vi "LDA_Align_PN_8 point.vi"(1 "Align Probe Using":enum16{"Green Beams", "Blue Beams"}(ring), 2 "Use Specification Beam Half-Angle":bool) -> (0 "Beam Data":T2={"Vg1 (Green 1 dir. vect.)"=[0.059117350659853476, -0.996541267827751, 0.05840068807144843], "Vg2  (Green 2 dir. vect.)"=[-0.05232536310393669, -0.9971561380468801, -0.054237373935992664], "Vb1 (Blue 1 dir. vect.)"=[-0.052923229613528855, -0.9969242065933935, 0.057803616456121795], "Vb2 (Blue 1 dir. vect.)"=[0.05971521716944564, -0.9967731992812374, -0.05364030232066602], "Porb (Orb XYZ posn. forced coplanar)"=[2201.0738225655555, -1199.3737231995547, 269.758310600838], "Porb (Orb XYZ posn. - allow skew)"=[2200.796256301178, -1199.3740953152687, 270.0329332816893], "Orb posn. uncertainty, +/- dx, dy, dz"=[0.13878313218879157, 0.00018605785703584843, 0.13731134042564008], "Vp (Actual Probe dir. vect)"=[0.003406702197773746, -0.9999920168246164, 0.0020882210543692924], "Yaw (deg)"=89.80480953887573, "Pitch (deg)"=0.11964634006213794, "In-Plane Roll (deg)"=45.305328966424156, "Beam Half Angle (deg)"=4.544091484248422, "B1 Close P11"=[0.0, 0.0, 0.0], "B1 Far P12"=[2158.01, -491.04, 229.28], "B2 Close P22"=[2158.01, -491.04, 229.28], "B2 Far P21"=[2158.01, -491.04, 229.28], "Projected Roll (deg)"=0.0, "Green Velocity Vector"=[0.0, 0.0, 0.0], "Blue Velocity Vector"=[0.0, 0.0, 0.0], "Probe is facing...."="-", "Calculation Method"=""} {"Vp (Actual Probe dir. vect)" format="%#_6f"; "Vg2  (Green 2 dir. vect.)" format="%#_6f"; "Vg1 (Green 1 dir. vect.)" format="%#_6f"})   [LabVIEW 2011]
uses:
  Controls/LDA_Beam_Cluster.ctl
  Gen Trav/Route mapping/Axis.ctl
  Controls/Tunnel_Coordinates.ctl
  Controls/User_Specific_mode.ctl
  Gen Trav/Trav_mode.ctl
  Globals/LDA_meas_global_1.vi
  Globals/Trav_pos_global.vi
panel:
  out "8 Peaked positions":dbl[][](array[numeric])
  out "Peakup up inputs":dbl[][](array[numeric])
  out "Fixed Axis":T1
  out "png folder":path
  out "Taught point names":string[](array[string])
  out "Taught Positions":dbl[][](array[numeric])
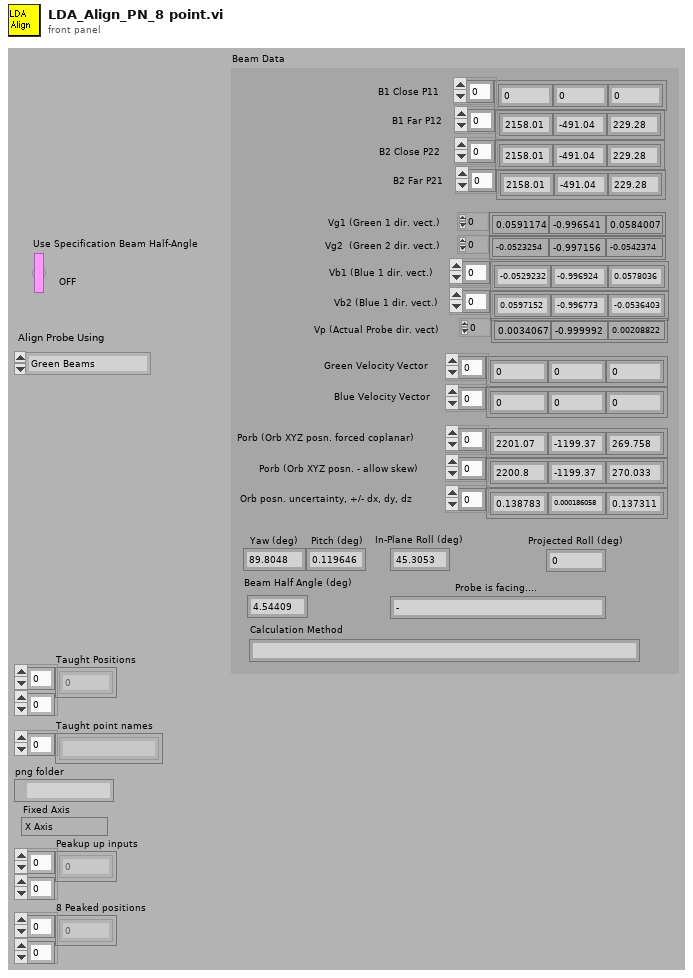
[diagram p1: front panel]
types:
  T1 = typedef "Axis.ctl" = enum16{"X Axis", "X Axis -ve", "Y Axis", "Y Axis -ve", "Z Axis", "Z Axis -ve"}
  T2 = typedef "LDA_Beam_Cluster.ctl" = cluster{"Vg1 (Green 1 dir. vect.)":dbl[], "Vg2  (Green 2 dir. vect.)":dbl[], "Vb1 (Blue 1 dir. vect.)":dbl[], "Vb2 (Blue 1 dir. vect.)":dbl[], "Porb (Orb XYZ posn. forced coplanar)":dbl[], "Porb (Orb XYZ posn. - allow skew)":dbl[], "Orb posn. uncertainty, +/- dx, dy, dz":dbl[], "Vp (Actual Probe dir. vect)":dbl[], "Yaw (deg)":dbl, "Pitch (deg)":dbl, "In-Plane Roll (deg)":dbl, "Beam Half Angle (deg)":dbl, "B1 Close P11":dbl[], "B1 Far P12":dbl[], "B2 Close P22":dbl[], "B2 Far P21":dbl[], "Projected Roll (deg)":dbl, "Green Velocity Vector":dbl[], "Blue Velocity Vector":dbl[], "Probe is facing....":string, "Calculation Method":string}
  T3 = typedef "Tunnel_Coordinates.ctl" = enum16{"Work in Tunnel Coordinates", "Work in Model Coordinates"}
  T4 = typedef "User_Specific_mode.ctl" = enum16{"Check VI only", "Run VI"}
  T5 = typedef "Trav_mode.ctl" = enum16{"Move traverse", "Read traverse position", "Teach Position"}
  T6 = enum16{"Load setup from excel file", "Save setup to excel file"}
  T7 = cluster{"second":i32, "minute":i32, "hour":i32, "day of month":i32, "month":i32, "year":i32, "day of week":i32, "day of year":i32, "is DST":i32}
  T8 = typedef "Multi_Run_Status.ctl" = enum16{"Continue", "Jump to Next Point", "Jump to Next Row", "Jump To Fall Back", "Terminate Run"}
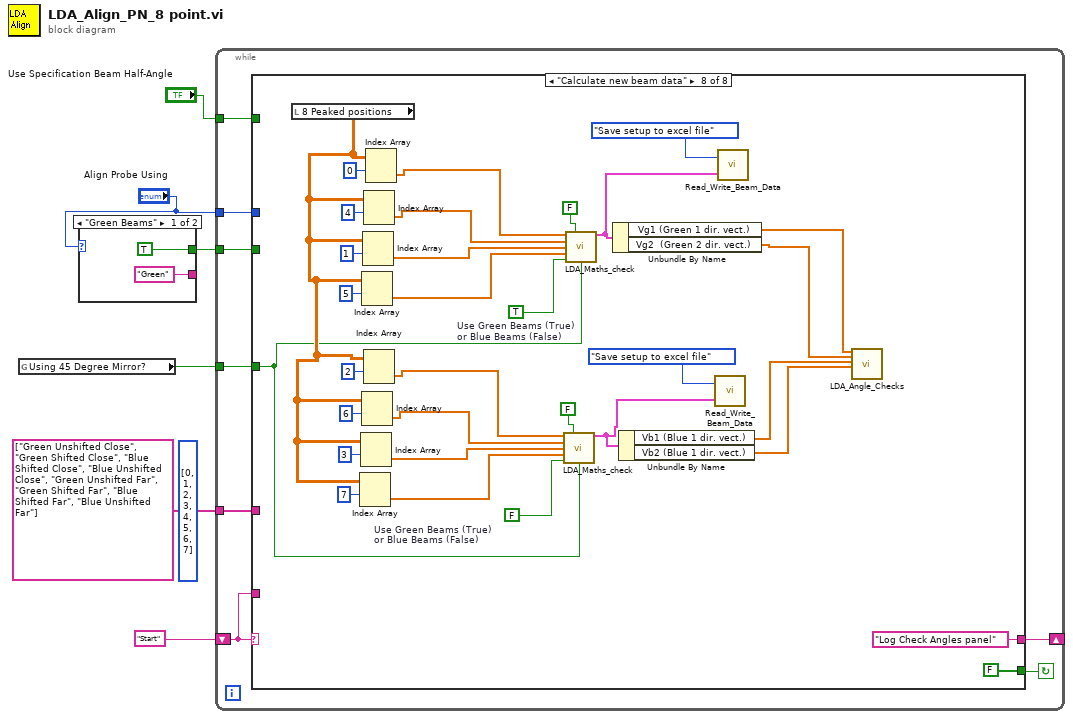
[diagram p0: block diagram]
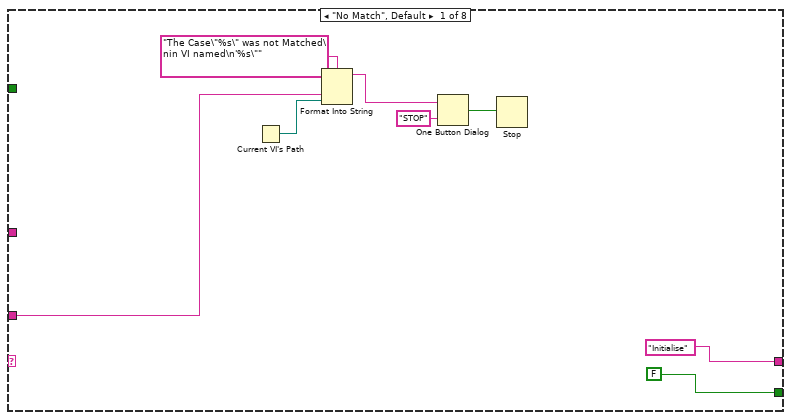
[diagram p2: hidden frame]
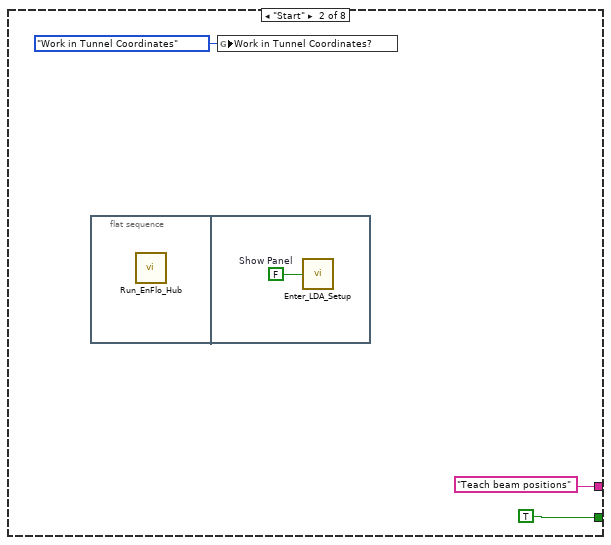
[diagram p3: hidden frame]
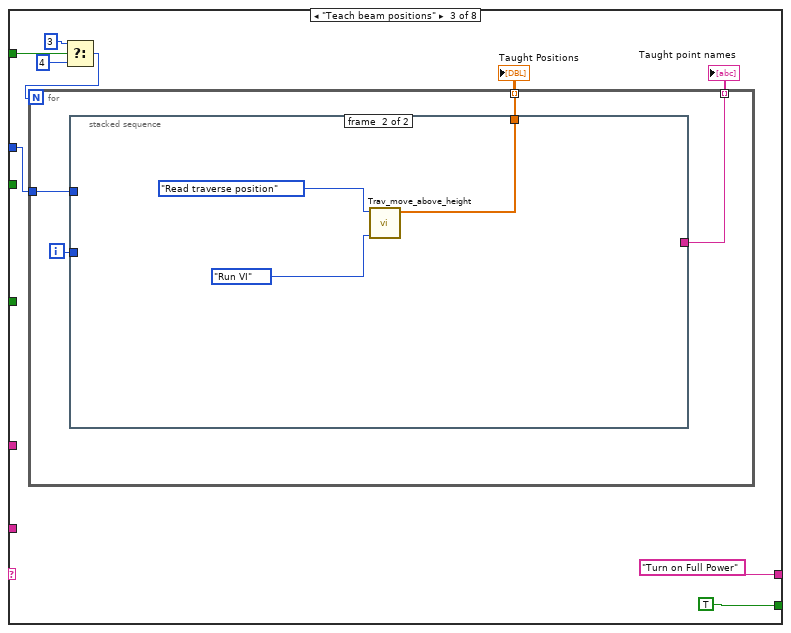
[diagram p4: hidden frame]
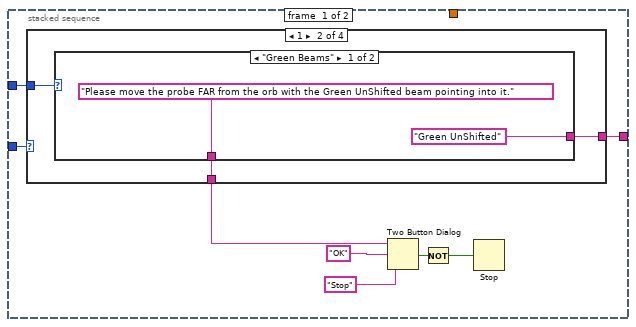
[diagram p5: hidden frame]
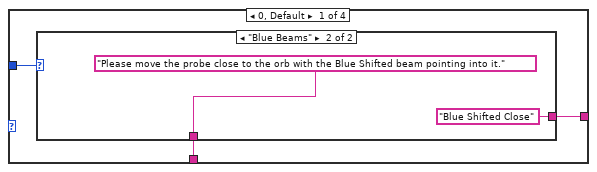
[diagram p6: hidden frame]
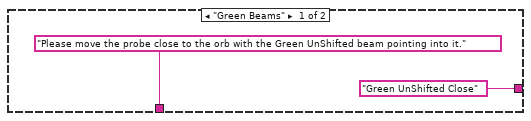
[diagram p7: hidden frame]
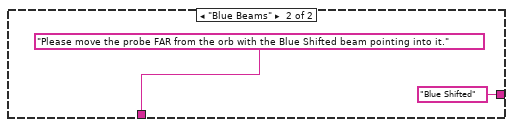
[diagram p8: hidden frame]
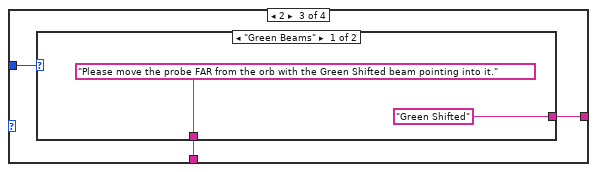
[diagram p9: hidden frame]
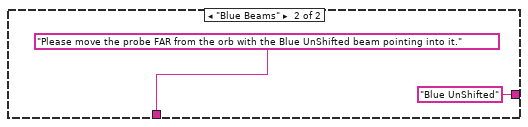
[diagram p10: hidden frame]
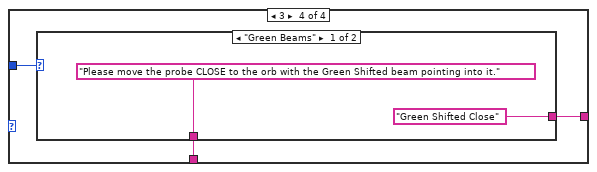
[diagram p11: hidden frame]
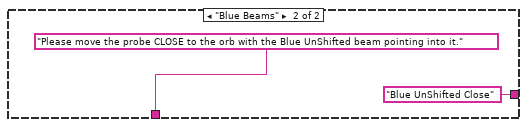
[diagram p12: hidden frame]
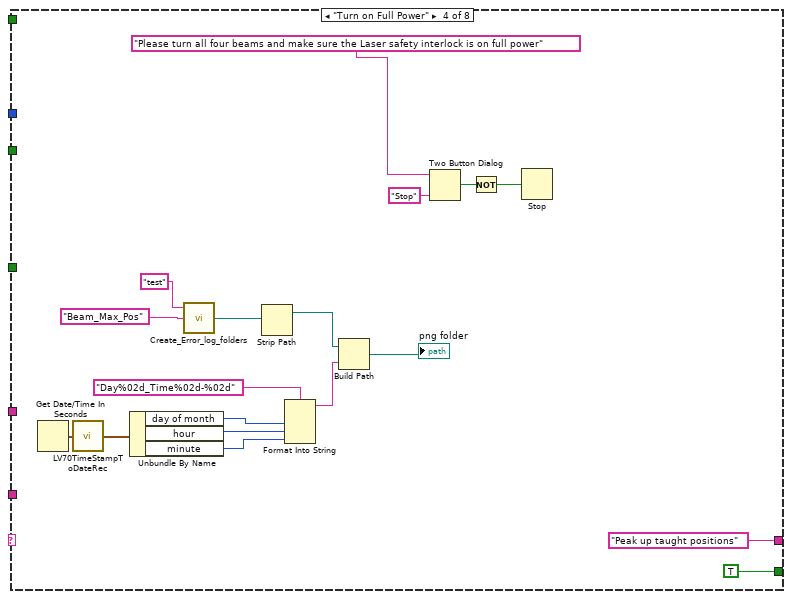
[diagram p13: hidden frame]
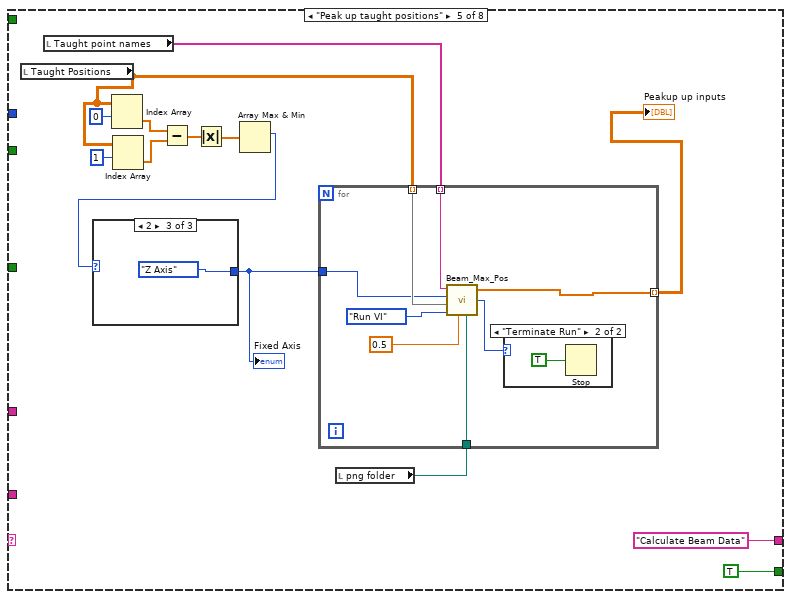
[diagram p14: hidden frame]
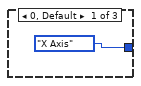
[diagram p15: hidden frame]
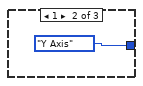
[diagram p16: hidden frame]
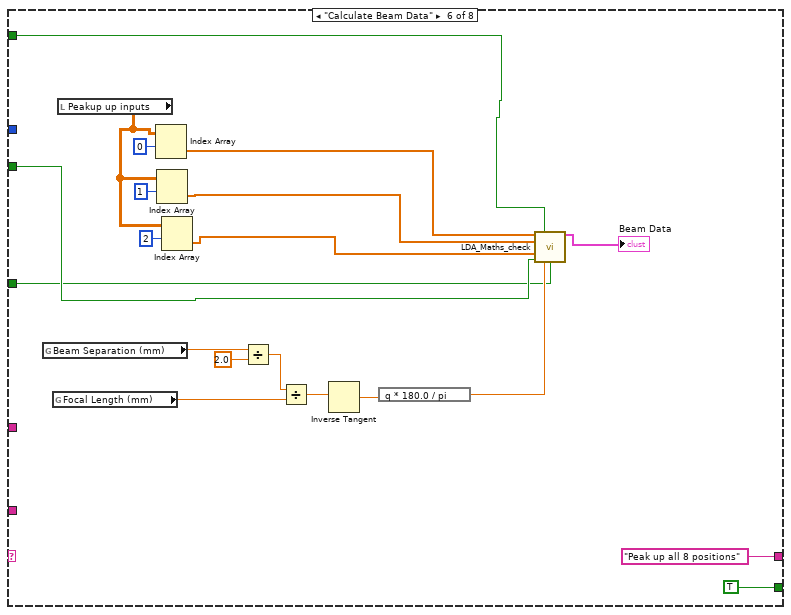
[diagram p18: hidden frame]
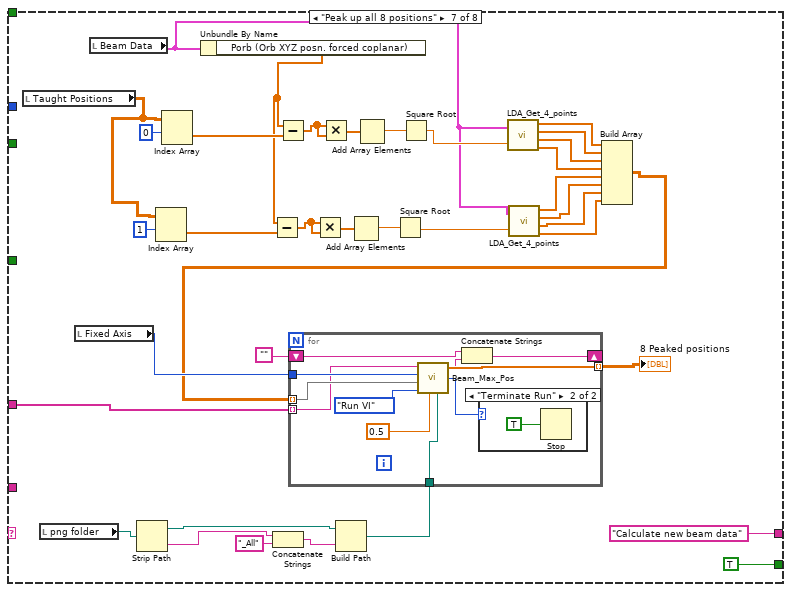
[diagram p19: hidden frame]
diagram:
  (unwired) i32[] [0, 1, 2, 3, 4, 5, 6, 7] ("appended array")
  n1 = global read "LDA_meas_global_1.vi" "Using 45 Degree Mirror?"() -> (w1:bool)
  n2 = case shown="\"Green Beams\"" "Align Probe Using" {
    tunnel: [TRUE FALSE] -> w3
    tunnel: ["Green" "Blue"] -> _
    frame "Green Beams" {
    }
    frame "Blue Beams" {
    }
  }
  n3 = while {
    shift-left: "Start" -> [w16]
    shift-right: [w17] -> _
    tunnel: "Align Probe Using" -> [w15]
    tunnel: "Use Specification Beam Half-Angle" -> [w14]
    tunnel: w3 -> [w13]
    tunnel: string[] ["Green Unshifted Close", "Green Shifted Close", "Blue Shifted Close", "Blue Unshifted Close", "Green Unshifted Far", "Green Shifted Far", "Blue Shifted Far", "Blue Unshifted Far"] ("appended array") -> [w12]
    tunnel: w1 -> [w11]
    stop <- w18 continue-if-true
    n4 = case shown="\"Calculate new beam data\"" w16 {
      tunnel: [FALSE TRUE TRUE TRUE TRUE TRUE TRUE FALSE] -> w18
      tunnel: ["Initialise" "Teach beam positions" "Turn on Full Power" "Peak up taught positions" "Calculate Beam Data" "Peak up all 8 positions" "Calculate new beam data" "Log Check Angles panel"] -> w17
      tunnel: w16 -> [w21 _ _ _ _ _ _ _]
      tunnel: w15 -> [_ _ w37 _ _ _ _ _]
      tunnel: w14 -> [_ _ w34 _ _ w144 _ _]
      tunnel: w13 -> [_ _ _ _ _ w143 _ _]
      tunnel: w12 -> [_ _ _ _ _ _ w149 _]
      tunnel: w11 -> [_ _ _ _ _ w127 _ w195]
      frame "No Match", Default {
        n5 = Current VI's Path() -> (path=w20:path)
        n6 = Format Into String(format string="The Case\"%s\" was not Matched\nin VI named\n'%s\"" ("Format String"), w21, w20) -> (resulting string=w24:string)  [unwired: 2 in, 1 out]
        n7 = One Button Dialog(message=w24, button name ("OK")="STOP") -> (true=w22:bool)
        n8 = Stop(stop? (T)=w22) -> ()
      }
      frame "Start" {
        n9 = flat-sequence {
          frame #0 {
            n10 = call "Run_EnFlo_Hub.vi"() -> ()  [unwired: 8 out]
          }
          frame #1 {
            w30 = FALSE  # Show Panel
            n11 = call "Enter_LDA_Setup.vi"("Show Panel"=w30) -> ()
          }
        }
        n12 = global write "Trav_pos_global.vi" "Work in Tunnel Coordinates?"(Tunnel_Coordinates."Work in Tunnel Coordinates" ("Work in Tunnel Coordinates?")) -> ()
      }
      frame "Teach beam positions" {
        n13 = Select(t=3, s=w34, f=4) -> (s? t:f=w33:i32)
        n14 = for {
          N: w33 -> [_]
          tunnel: [w43] -> w32 mode=indexing
          tunnel: w37 -> [w42]
          tunnel: [w41] -> w31 mode=indexing
          i -> [w40]
          n15 = stacked-sequence {
            tunnel: [_ w80] -> w43
            tunnel: w42 -> [w50 _]
            tunnel: [w45 _] -> w41
            tunnel: w40 -> [w44 _]
            frame #0 {
              n16 = case shown="1" w44 {
                tunnel: [w54 w61 w68 w75] -> w51
                tunnel: w50 -> [w53 w60 w67 w74]
                tunnel: [w52 w59 w66 w73] -> w45
                frame 0, Default {
                  n17 = case shown="\"Blue Beams\"" w53 {
                    tunnel: ["Please move the probe close to the orb with the Green UnShifted beam pointing into it." ("message") "Please move the probe close to the orb with the Blue Shifted beam pointing into it." ("message")] -> w54
                    tunnel: ["Green UnShifted Close" "Blue Shifted Close"] -> w52
                    frame "Green Beams" {
                    }
                    frame "Blue Beams" {
                    }
                  }
                }
                frame 1 {
                  n18 = case shown="\"Green Beams\"" w60 {
                    tunnel: ["Please move the probe FAR from the orb with the Green UnShifted beam pointing into it." ("message") "Please move the probe FAR from the orb with the Blue Shifted beam pointing into it." ("message")] -> w61
                    tunnel: ["Green UnShifted" "Blue Shifted"] -> w59
                    frame "Green Beams" {
                    }
                    frame "Blue Beams" {
                    }
                  }
                }
                frame 2 {
                  n19 = case shown="\"Green Beams\"" w67 {
                    tunnel: ["Please move the probe FAR from the orb with the Green Shifted beam pointing into it." ("message") "Please move the probe FAR from the orb with the Blue UnShifted beam pointing into it." ("message")] -> w68
                    tunnel: ["Green Shifted" "Blue UnShifted"] -> w66
                    frame "Green Beams" {
                    }
                    frame "Blue Beams" {
                    }
                  }
                }
                frame 3 {
                  n20 = case shown="\"Green Beams\"" w74 {
                    tunnel: ["Please move the probe CLOSE to the orb with the Green Shifted beam pointing into it." ("message") "Please move the probe CLOSE to the orb with the Blue UnShifted beam pointing into it." ("message")] -> w75
                    tunnel: ["Green Shifted Close" "Blue UnShifted Close"] -> w73
                    frame "Green Beams" {
                    }
                    frame "Blue Beams" {
                    }
                  }
                }
              }
              n21 = Two Button Dialog(message=w51, 1:"Stop" ("F button name (\"Cancel\")"), 2:"OK" ("T button name (\"OK\")")) -> (T button?=w47:bool)
              n22 = Not(x=w47) -> (.not. x?=w46:bool)
              n23 = Stop(stop? (T)=w46) -> ()
            }
            frame #1 {
              n24 = call "Trav_move_above_height.vi"("Simulate/Run"=User_Specific_mode."Run VI", "Mode"=Trav_mode."Read traverse position") -> ("Trav Position achieved"=w80:dbl[])  [unwired: 5 in, 4 out]
            }
          }
        }
        "Taught Positions" <- w32
        "Taught point names" <- w31
      }
      frame "Turn on Full Power" {
        n25 = Get Date/Time In Seconds() -> (seconds since 1Jan1904=w83:timestamp)
        n26 = call <vilib>:"LV70TimeStampToDateRec.vi"("time stamp"=w83) -> ("date time rec"=w92:T7)
        n27 = Unbundle By Name(w92) -> ("day of month"=w89:i32, "hour"=w90:i32, "minute"=w91:i32)
        n28 = call "Create_Error_log_folders.vi"("Log Folder"="Beam_Max_Pos" ("name or relative path"), "Log Filename"="test") -> ("Server copy Location"=w84:path)  [unwired: 1 in, 2 out]
        n29 = Strip Path(path=w84) -> (stripped path=w93:path)  [unwired: 1 out]
        n30 = Format Into String(format string="Day%02d_Time%02d-%02d", w89, w90, w91) -> (resulting string=w94:string)  [unwired: 2 in, 1 out]
        n31 = Build Path(base path=w93, name or relative path=w94) -> (appended path=→"png folder":path)
        n32 = Two Button Dialog(message="Please turn all four beams and make sure the Laser safety interlock is on full power", 1:"Stop" ("F button name (\"Cancel\")")) -> (T button?=w98:bool)  [unwired: 1 out]
        n33 = Not(x=w98) -> (.not. x?=w99:bool)
        n34 = Stop(stop? (T)=w99) -> ()
      }
      frame "Peak up taught positions" {
        n35 = local read "Taught Positions"() -> (w105:dbl[][])
        n36 = local read "Taught point names"() -> (w104:string[])
        n37 = Index Array(array=w105, index (row)=0) -> (element=w108:dbl[])  [unwired: 1 in]
        n38 = Index Array(array=w105, index (row)=1) -> (element=w109:dbl[])  [unwired: 1 in]
        n39 = Subtract(x=w108, y=w109) -> (x-y=w110:dbl[])
        n40 = Absolute Value(x=w110) -> (abs(x)=w111:dbl[])
        n41 = Array Max & Min(array=w111) -> (max index (indices)=w112:i32)  [unwired: 3 out]
        n42 = case shown="2" w112 {
          tunnel: [Axis."X Axis" ("Fixed Axis") Axis."Y Axis" ("Fixed Axis") Axis."Z Axis" ("Fixed Axis")] -> w103
          frame 0, Default {
          }
          frame 1 {
          }
          frame 2 {
          }
        }
        "Fixed Axis" <- w103
        n43 = local read "png folder"() -> (w102:path)
        n44 = for {
          tunnel: w104 -> [w125] mode=indexing
          tunnel: w105 -> [w124] mode=indexing
          tunnel: w103 -> [w122]
          tunnel: w102 -> [w121]
          tunnel: [w120] -> w101 mode=indexing
          n45 = call "Beam_Max_Pos.vi"("Picture Log"=w121, "Search Step (mm)"=0.5, "Mode"=User_Specific_mode."Run VI", "Starting Position"=w124, "Fixed Axis"=w122, "Beam Name"=w125) -> ("Status"=w118:T8, "Beam maxima"=w120:dbl[])  [unwired: 1 in, 2 out]
          n46 = case shown="\"Terminate Run\"" w118 {
            frame "Continue", Default {
            }
            frame "Terminate Run" {
              n47 = Stop(stop? (T)=TRUE) -> ()
            }
          }
        }
        "Peakup up inputs" <- w101
      }
      frame "Calculate Beam Data" {
        n48 = global read "LDA_meas_global_1.vi" "Beam Separation (mm)"() -> (w130:dbl)
        n49 = global read "LDA_meas_global_1.vi" "Focal Length (mm)"() -> (w133:dbl)
        n50 = local read "Peakup up inputs"() -> (w136:dbl[][])
        n51 = Index Array(array=w136, index (row)=0) -> (element=w140:dbl[])  [unwired: 1 in]
        n52 = Index Array(array=w136, index (row)=1) -> (element=w141:dbl[])  [unwired: 1 in]
        n53 = Index Array(array=w136, index (row)=2) -> (element=w142:dbl[])  [unwired: 1 in]
        n54 = Divide(x=w130, y=2.0) -> (x/y=w132:dbl)
        n55 = Divide(x=w132, y=w133) -> (x/y=w135:dbl)
        n56 = Inverse Tangent(1:w135) -> (0:w134:dbl)
        n57 = expression code="q * 180.0 / pi"(w134) -> (w129:dbl)
        n58 = call "LDA_Maths_check.vi"("B1 Close P11"=w140, "Use Specification Beam Half-Angle"=w144, "B1 Far P12"=w141, "B2 Far P21"=w142, "Use Green Beams (True) or Blue Beams (False)"=w143, "Beam Half-Angle (deg)"=w129, "Using 45 Degree Mirror?"=w127) -> ("Beam Data"=→"Beam Data":T2)  [unwired: 8 out]
      }
      frame "Peak up all 8 positions" {
        n59 = local read "Taught Positions"() -> (w170:dbl[][])
        n60 = local read "png folder"() -> (w161:path)
        n61 = local read "Fixed Axis"() -> (w162:T1)
        n62 = local read "Beam Data"() -> (w168:T2)
        n63 = Strip Path(path=w161) -> (stripped path=w157:path, name=w160:string)
        n64 = Index Array(array=w170, index (row)=1) -> (element=w171:dbl[])  [unwired: 1 in]
        n65 = Index Array(array=w170, index (row)=0) -> (element=w180:dbl[])  [unwired: 1 in]
        n66 = Unbundle By Name(w168) -> ("Porb (Orb XYZ posn. forced coplanar)"=w148:dbl[])
        n67 = Subtract(x=w148, y=w171) -> (x-y=w175:dbl[])
        n68 = Concatenate Strings(w160, "_All" ("string")) -> (w158:string)
        n69 = Subtract(x=w148, y=w180) -> (x-y=w176:dbl[])
        n70 = Multiply(x=w175, y=w175) -> (x*y=w174:dbl[])
        n71 = Multiply(x=w176, y=w176) -> (x*y=w177:dbl[])
        n72 = Build Path(base path=w157, name or relative path=w158) -> (appended path=w147:path)
        n73 = Add Array Elements(numeric array=w174) -> (sum=w173:dbl)
        n74 = Add Array Elements(numeric array=w177) -> (sum=w178:dbl)
        n75 = Square Root(x=w173) -> (sqrt(x)=w167:dbl)
        n76 = Square Root(x=w178) -> (sqrt(x)=w169:dbl)
        n77 = call "LDA_Get_4_points.vi"("Beam Data"=w168, "L, Probe-Normal Distance"=w169) -> ("Pg1"=w166:dbl[], "Pg2"=w165:dbl[], "Pb1"=w164:dbl[], "Pb2"=w163:dbl[])
        n78 = call "LDA_Get_4_points.vi"("Beam Data"=w168, "L, Probe-Normal Distance"=w167) -> ("Pg1"=w154:dbl[], "Pg2"=w153:dbl[], "Pb1"=w155:dbl[], "Pb2"=w156:dbl[])
        n79 = Build Array(w166, w165, w164, w163, w154, w153, w155, w156) -> (w152:dbl[][])
        n80 = for {
          tunnel: w147 -> [w192]
          tunnel: [w191] -> w150 mode=indexing
          shift-right: [w188] -> _
          shift-left: "" -> [w190]
          tunnel: w152 -> [w185] mode=indexing
          tunnel: w162 -> [w184]
          tunnel: w149 -> [w183] mode=indexing
          n81 = call "Beam_Max_Pos.vi"("Picture Log"=w192, "Search Step (mm)"=0.5, "Mode"=User_Specific_mode."Run VI", "Starting Position"=w185, "Fixed Axis"=w184, "Beam Name"=w183) -> ("Status"=w186:T8, "Beam maxima"=w191:dbl[], "Message"=w189:string)  [unwired: 1 in, 1 out]
          n82 = Concatenate Strings(w190, w189) -> (w188:string)
          n83 = case shown="\"Terminate Run\"" w186 {
            frame "Continue", Default {
            }
            frame "Terminate Run" {
              n84 = Stop(stop? (T)=TRUE) -> ()
            }
          }
        }
        "8 Peaked positions" <- w150
      }
      frame "Calculate new beam data" {
        w208 = FALSE  # Use Green Beams (True) or Blue Beams (False)
        w225 = TRUE  # Use Green Beams (True) or Blue Beams (False)
        n85 = local read "8 Peaked positions"() -> (w206:dbl[][])
        n86 = Index Array(array=w206, index (row)=7) -> (element=w216:dbl[])  [unwired: 1 in]
        n87 = Index Array(array=w206, index (row)=3) -> (element=w215:dbl[])  [unwired: 1 in]
        n88 = Index Array(array=w206, index (row)=5) -> (element=w217:dbl[])  [unwired: 1 in]
        n89 = Index Array(array=w206, index (row)=6) -> (element=w214:dbl[])  [unwired: 1 in]
        n90 = Index Array(array=w206, index (row)=1) -> (element=w218:dbl[])  [unwired: 1 in]
        n91 = Index Array(array=w206, index (row)=4) -> (element=w219:dbl[])  [unwired: 1 in]
        n92 = Index Array(array=w206, index (row)=2) -> (element=w210:dbl[])  [unwired: 1 in]
        n93 = Index Array(array=w206, index (row)=0) -> (element=w223:dbl[])  [unwired: 1 in]
        n94 = call "LDA_Maths_check.vi"("B1 Close P11"=w210, "Use Specification Beam Half-Angle"=FALSE, "B1 Far P12"=w214, "B2 Close P22"=w215, "B2 Far P21"=w216, "Use Green Beams (True) or Blue Beams (False)"=w208, "Using 45 Degree Mirror?"=w195) -> ("Beam Data"=w196:T2)  [unwired: 1 in, 7 out]
        n95 = call "LDA_Maths_check.vi"("B1 Close P11"=w223, "Use Specification Beam Half-Angle"=FALSE, "B1 Far P12"=w219, "B2 Close P22"=w218, "B2 Far P21"=w217, "Use Green Beams (True) or Blue Beams (False)"=w225, "Using 45 Degree Mirror?"=w195) -> ("Beam Data"=w199:T2)  [unwired: 1 in, 7 out]
        n96 = Unbundle By Name(w199) -> ("Vg1 (Green 1 dir. vect.)"=w205:dbl[], "Vg2  (Green 2 dir. vect.)"=w204:dbl[])
        n97 = Unbundle By Name(w196) -> ("Vb1 (Blue 1 dir. vect.)"=w203:dbl[], "Vb2 (Blue 1 dir. vect.)"=w202:dbl[])
        n98 = call "Read_Write_Beam_Data.vi"("Beam Data In"=w196, "Mode"=T6."Save setup to excel file") -> ()  [unwired: 1 out]
        n99 = call "Read_Write_Beam_Data.vi"("Beam Data In"=w199, "Mode"=T6."Save setup to excel file") -> ()  [unwired: 1 out]
        n100 = call "LDA_Angle_Checks.vi"("Vg1"=w205, "Vg2"=w204, "Vb1"=w203, "Vb2"=w202) -> ()  [unwired: 16 out]
      }
    }
  }
